vi "Time Estimate String.vi"(8 "error in (no error)":errorcluster, 9 "Time":dbl[unit], 10 "Steps":dbl) -> (0 "error out":errorcluster, 2 "Time Estimate String":string)   [LabVIEW 2017]
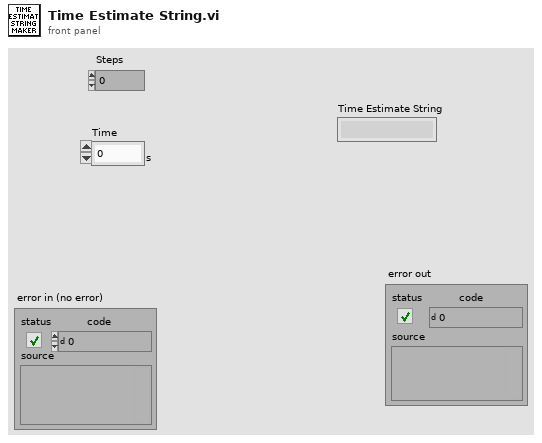
[diagram p1: front panel]
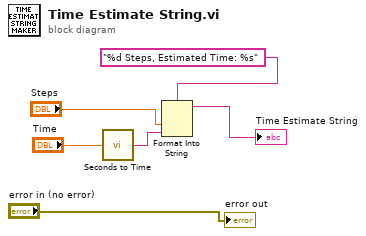
[diagram p0: block diagram]
diagram:
  n1 = call "Seconds to Time.vi"("Seconds"="Time") -> ("Time"=w5:string)
  n2 = Format Into String(format string="%d Steps, Estimated Time: %s", "Steps", w5) -> (resulting string=→"Time Estimate String":string)  [unwired: 2 in, 1 out]
  "error out" <- "error in (no error)"
